vi "IncrementTap.vi"(8 "Reset?":bool, 11 "Settings":T1={"Name of test"="", "Date"=timestamp(0 s since 1904-01-01), "Location"="", "Template"="", "Soundcard"="", "resolution"=32, "Sampling rate"=48000, "Ch1 Gain "=25.0, "Ch2 Gain"=10.0, "Sample time (s)"=0.3, "Pre-trigger (s)"=0.01, "Hammer Threshold"=10.0, "Positions"=12, "Taps/Position"=5, "Set Names"="", "Freq resolution"=10.0, "Hammer cutoff"=0.0, "Mic cutoff"=0.0, "Double bounce "=0.0, "Hammer Cal"=10.0, "dB Offset"=0.0, "Accel Cal"=10.0, "Vibrometer Cal"=0.0, "Mic Cal"=0.0, "Output"=2, "Voltage Cal"=1.0, "Vibrometer Port"="ASRL27::INSTR", "Range"=4, "High Pass"=2, "Bandwidth"=4, "X Range"=[], "Y Range"=[], "dB Spread"=0.0, "Trigger"=0, "Ch_1"=25, "Ch_2"=25, "flip?"=FALSE, "60Hz"=FALSE, "Time offset"=0.0, "Piezo Cal"=1.0, "Default Notes"=""} {"Ch_2" min=1 step=1; "Ch_1" min=1 max=100 step=1; "Trigger" items=["Hammer (force)", "Self-tap", "Spacebar"]; "Bandwidth" items=["1 kHz"=1, "5 kHz"=5, "10 kHz"=10, "25 kHz"=25, "50 kHz"=50, "100 kHz"=100]; "High Pass" items=["Off", "13 Hz", "104 Hz"]; "Range" items=["10 mm/s"=1, "20 mm/s"=2, "50 mm/s"=5, "100 mm/s"=10, "200 mm/s"=20, "500 mm/s"=50, "1 m/s"=100, "2 m/s"=200]; "Output" items=["Accelerometer", "Speed (from acceleration)", "Microphone", "Vibrometer", "Piezo"]; "Voltage Cal" format="%#_13g"; "Ch2 Gain" format="%#_13g"; "Ch1 Gain" format="%#_13g"; "Double bounce" min=0.0; "Mic cutoff" min=0.0 format="%#_4g"; "Hammer cutoff" min=0.0 format="%#_4g"; "Freq resolution" min=0.0; "Pre-trigger (s)" format="%#_13g"; "Date" format="%<%H:%M\n%d/%m/%y>T"; "resolution" items=["16 bit"=16, "24 bit"=24, "32 bit"=32]; "Sampling rate" items=["22050 samp/s"=22050, "44100 samp/s"=44100, "48000 samp/s"=48000]}) -> (0 "Done?":bool, 1 "Last Data Set":path, 2 "files":i32, 3 "New File":string, 4 "Location":cluster{"Set":i16, "Position":i16, "Tap":i16}, 6 "Next Location":cluster{"Set":i16, "Position":i16, "Tap":i16})   [LabVIEW 2022 SP3]
uses:
  PreferencesControl.ctl
panel:
  # "Hz"
  # "dB"
  # "dB"
  # "sec"
  # "sec"
  # "mV/Pa"
  # "mV/m/s2"
  # "mV/mm/s"
  # "V/N"
  # "sec"
  # "sec"
  # "mV/N"
  # "a.u."
  # "a.u."
  # "sec"
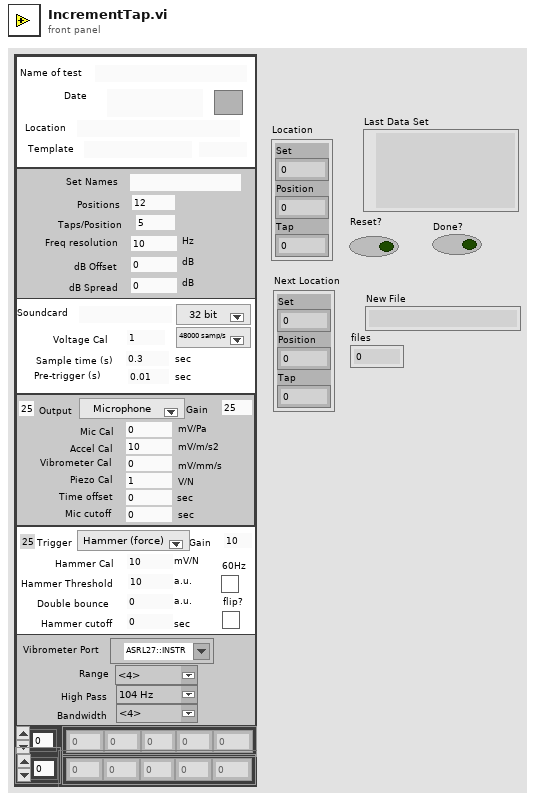
[diagram p1: front panel]
types:
  T1 = typedef "PreferencesControl.ctl" = cluster{"Name of test":string, "Date":timestamp, "Location":string, "Template":string, "Soundcard":string, "resolution":u16, "Sampling rate":u16, "Ch1 Gain ":dbl, "Ch2 Gain":dbl, "Sample time (s)":dbl, "Pre-trigger (s)":dbl, "Hammer Threshold":dbl, "Positions":i16, "Taps/Position":i16, "Set Names":string, "Freq resolution":dbl, "Hammer cutoff":dbl, "Mic cutoff":dbl, "Double bounce ":dbl, "Hammer Cal":dbl, "dB Offset":dbl, "Accel Cal":dbl, "Vibrometer Cal":dbl, "Mic Cal":dbl, "Output":u16, "Voltage Cal":dbl, "Vibrometer Port":refnum<visa-resource-name>, "Range":u16, "High Pass":u16, "Bandwidth":u16, "X Range":cluster{"Minimum":dbl, "Maximum":dbl, "Increment":dbl, "Minor Increment":dbl, "Start":dbl}[], "Y Range":cluster{"Minimum":dbl, "Maximum":dbl, "Increment":dbl, "Minor Increment":dbl, "Start":dbl}[], "dB Spread":dbl, "Trigger":u16, "Ch_1":u8, "Ch_2":u8, "flip?":bool, "60Hz":bool, "Time offset":dbl, "Piezo Cal":dbl, "Default Notes":string}
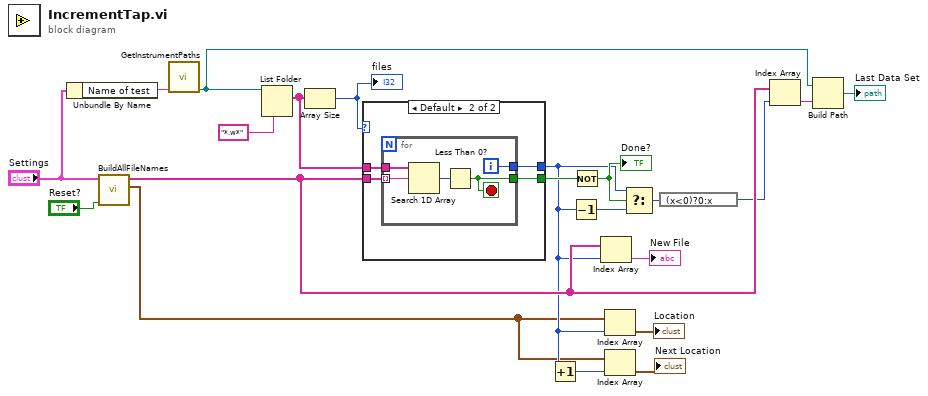
[diagram p0: block diagram]
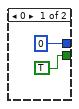
[diagram p2: hidden frame]
diagram:
  n1 = Unbundle By Name("Settings") -> ("Name of test"=w16:string)
  n2 = call "BuildAllFileNames.vi"("Reset?"="Reset?", "Settings"="Settings") -> ("Info"=w2:cluster{i32, i32, i32}[], "File Names"=w13:string[])  [unwired: 8 in]
  n3 = call "GetInstrumentPaths.vi"("Instrument"=w16) -> ("Path To Raw Folder"=w11:path)  [unwired: 6 in, 4 out]
  n4 = List Folder(path=w11, pattern="*.w*") -> (filenames=w14:string[])  [unwired: 2 in, 3 out]
  n5 = Array Size(array=w14) -> (size(s)=w15:i32)
  "files" <- w15
  n6 = case shown="Default" w15 {
    tunnel: w14 -> [_ w27]
    tunnel: [TRUE w26] -> w8
    tunnel: w13 -> [_ w25]
    tunnel: [0 w24] -> w4
    frame 0 {
    }
    frame Default {
      n7 = for {
        tunnel: w27 -> [w32]
        tunnel: w25 -> [w29] mode=indexing
        tunnel: [w30] -> w26
        tunnel: [w28] -> w24
        i -> [w28]
        stop <- w30 stop-if-true
        n8 = Search 1D Array(1D array=w32, element=w29) -> (index of element=w31:i32)  [unwired: 1 in]
        n9 = Less Than 0?(x=w31) -> (x < 0?=w30:bool)
      }
    }
  }
  n10 = Increment(x=w4) -> (x+1=w3:i32)
  n11 = Decrement(x=w4) -> (x-1=w10:i32)
  n12 = Not(x=w8) -> (.not. x?=w21:bool)
  "Done?" <- w21
  n13 = Index Array(array=w13, index=w4) -> (element=→"New File":string)
  n14 = Index Array(array=w2, index=w4) -> (element=→"Location":cluster{i32, i32, i32})
  n15 = Index Array(array=w2, index=w3) -> (element=→"Next Location":cluster{i32, i32, i32})
  n16 = Select(t=w4, s=w21, f=w10) -> (s? t:f=w9:i32)
  n17 = expression code="(x<0)?0:x"(w9) -> (w5:i32)
  n18 = Index Array(array=w13, index=w5) -> (element=w12:string)
  n19 = Build Path(base path=w11, name or relative path=w12) -> (appended path=→"Last Data Set":path)
